vi "DAC Init Results.vi"(8 "error in":errorcluster, 9 "Log Details?":bool, 10 "tdms file":refnum<k34>, 11 "DAC LN2 Temp in":refnum<class "DAC LN2 Temp.lvclass">) -> (0 "error out":errorcluster, 2 "tdms file out":refnum<k34>)   [LabVIEW 2019, in "DAC.lvlib" / "DAC LN2 Temp.lvclass"]
uses:
  DAC LN2 Temp.lvclass
  DAC.lvclass
  C:/Users/wg/Documents/LV_Projects/test-stand/App/DAC/DAC.lvclass
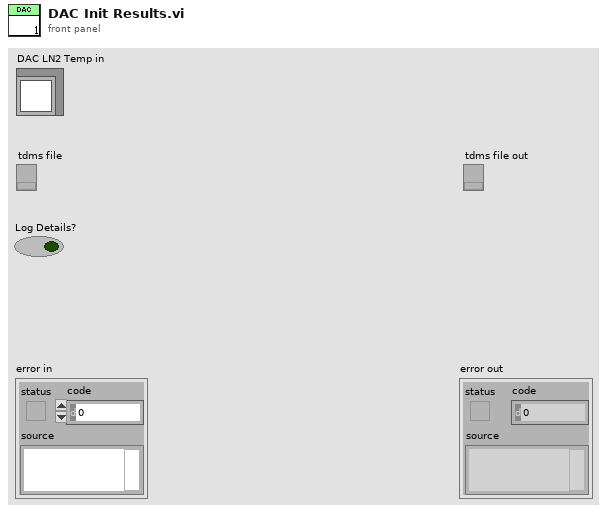
[diagram p1: front panel]
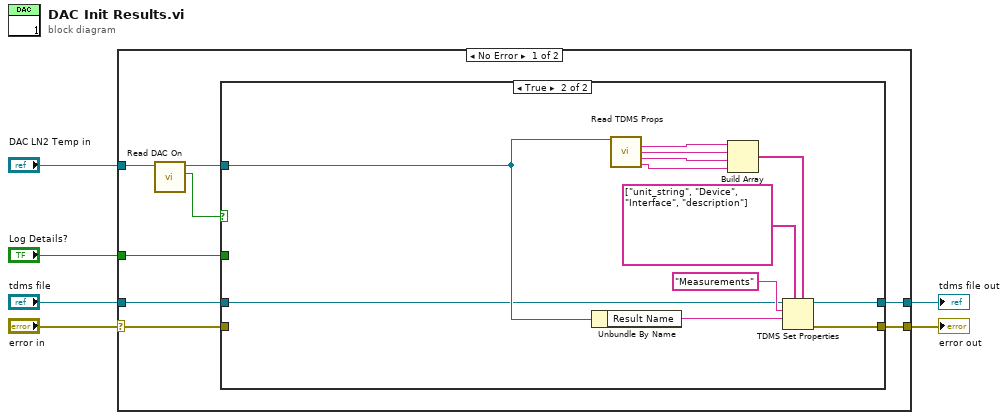
[diagram p0: block diagram]
diagram:
  n1 = case shown="No Error" "error in" {
    selector: "error in" -> [w10 w30]
    tunnel: [w7 w30] -> w6
    tunnel: "DAC LN2 Temp in" -> [w14 _]
    tunnel: "tdms file" -> [w11 w29]
    tunnel: [w8 w29] -> w5
    tunnel: "Log Details?" -> [w9 _]
    frame No Error {
      n2 = call "Read DAC On.vi"("DAC in"=w14) -> ("DAC On"=w12:bool, "DAC out"=w13:refnum<class "DAC LN2 Temp.lvclass">)  [unwired: 8 in, 1 out]
      n3 = case shown="True" w12 {
        tunnel: w11 -> [w15 w17]
        tunnel: [w15 w20] -> w8
        tunnel: [w16 w18] -> w7
        tunnel: w13 -> [_ w19]
        tunnel: w10 -> [w16 _]
        tunnel: w9 -> [_ _]
        frame False {
        }
        frame True {
          n4 = Unbundle By Name(w19) -> ("Result Name"=w27:string)
          n5 = call "Read TDMS Props.vi"("DAC in"=w19) -> ("Result Unit"=w26:string, "DAC Device"=w25:string, "DAC IO"=w24:string, "DAC Description"=w23:string)  [unwired: 10 in, 1 out]
          n6 = Build Array(w26, w25, w24, w23) -> (w21:string[])
          n7 = TDMS Set Properties(5:w21, 7:string[] ["unit_string", "Device", "Interface", "description"] ("property names"), 9:w27, 10:"Measurements" ("group name in (Untitled)"), 11:w17) -> (0:w18:errorcluster, 3:w20:refnum<k34>)  [unwired: 1 in, 2 out]
        }
      }
    }
    frame Error {
    }
  }
  "error out" <- w6
  "tdms file out" <- w5
